vi "Send Write DAQ Configuration .vi"(7 "Message Priority (Normal)":T1=enum."Normal", 8 "error in (no error)":errorcluster, 10 "DAQ Configuration":refnum<vi>, 11 "Message Enqueuer":refnum<class "Message Enqueuer.lvclass">) -> (0 "error out":errorcluster, 3 "Message Enqueuer out":refnum<class "Message Enqueuer.lvclass">)   [LabVIEW 2023, in "GUI.lvlib" / "Settings.lvlib" / "Write DAQ Configuration  Msg.lvclass"]
doc: "This VI sends the message to an actor."
uses:
  Write DAQ Configuration  Msg.lvclass
  Write DAQ Configuration  Msg.lvclass/Write DAQ Configuration  Msg.ctl
  <vilib>/ActorFramework/Message Enqueuer/Message Enqueuer.lvclass
  C:/Program Files/National Instruments/LabVIEW 2023/vi.lib/ActorFramework/Message/Message.lvclass
  D:/eDCU LTT/VT LTT Project/Source Code/GUI/Actor/Settings/Settings Messages/Write DAQ Configuration  Msg/Write DAQ Configuration  Msg.lvclass
  <vilib>/ActorFramework/Message Enqueuer/Message Priority.ctl
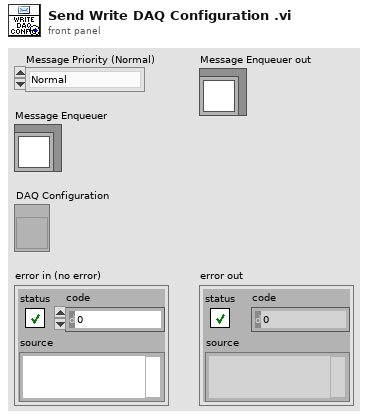
[diagram p1: front panel]
types:
  T1 = typedef "Actor Framework.lvlib/Message Enqueuer.lvclass/Message Priority.ctl" = enum16{"Low", "Normal", "High"}
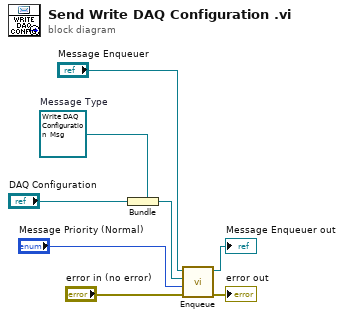
[diagram p0: block diagram]
diagram:
  w5 = refnum<class "Write DAQ Configuration  Msg.lvclass"> refnum  # Message Type
  n1 = Bundle(cluster=w5, "DAQ Configuration") -> (w4:refnum<class "Write DAQ Configuration  Msg.lvclass">)
  n2 = call <vilib>:"Enqueue.vi"("error in (no error)"="error in (no error)", "Message Priority (Normal)"="Message Priority (Normal)", "Message"=w4, "Message Enqueuer in"="Message Enqueuer") -> ("error out"=→"error out":errorcluster, "Message Enqueuer in"=→"Message Enqueuer out":refnum<class "Message Enqueuer.lvclass">)  [unwired: 6 in]
